vi "Retrieve Category SubPanel Information.vi"(8 "error in (no error)":errorcluster, 10 "ListBox Selection":i32, 11 "Configuration in":refnum<class "Configuration.lvclass">) -> (0 "error out":errorcluster, 1 "Help Text":string, 2 "VI Refnum":refnum<vi>, 3 "Configuration Out":refnum<class "Configuration.lvclass">)   [LabVIEW 2017, in "Configuration.lvlib" / "Configuration.lvclass"]
uses:
  Configuration.lvclass
  Configuration.lvclass/Configuration.ctl
  Data Retrieved by Lookup Table.ctl
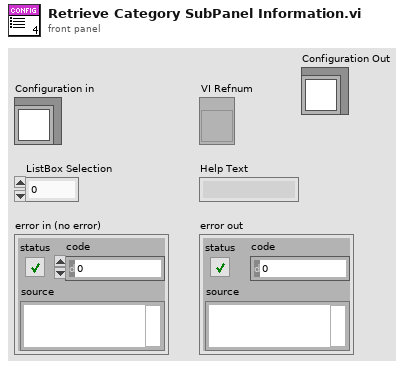
[diagram p1: front panel]
types:
  T1 = typedef "Configuration.lvlib/Configuration.lvclass/Data Retrieved by Lookup Table.ctl" = cluster{"VI Refnum":refnum<vi>, "Help Text":string}
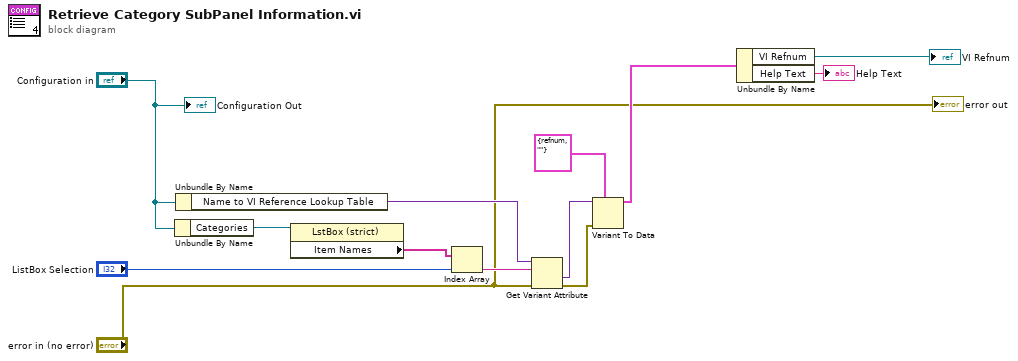
[diagram p0: block diagram]
diagram:
  n1 = Unbundle By Name("Configuration in") -> ("Categories"=w3:refnum<vi>)
  n2 = Unbundle By Name("Configuration in") -> ("Name to VI Reference Lookup Table"=w4:variant)
  n3 = property on="Property Node" class="LstBox (strict)"(reference=w3) -> ("Item Names"=w2:string[])  [unwired: 1 in, 2 out]
  n4 = Index Array(array=w2, index="ListBox Selection") -> (element=w5:string)
  n5 = Get Variant Attribute(Variant=w4, name=w5, error in="error in (no error)") -> (value=w6:variant, error out=w7:errorcluster)  [unwired: 1 in, 2 out]
  n6 = Variant To Data(error in=w7, type=T1 {"VI Refnum"=refnum, "Help Text"=""} ("output cluster"), Variant=w6) -> (data=w11:T1)  [unwired: 1 out]
  n7 = Unbundle By Name(w11) -> ("VI Refnum"=→"VI Refnum":refnum<vi>, "Help Text"=→"Help Text":string)
  "error out" <- "error in (no error)"
  "Configuration Out" <- "Configuration in"
